vi "Log Level.vi"(8 "error in (no error)":errorcluster, 11 "Configuration.Level":T1) -> (0 "error out":errorcluster)   [LabVIEW 2016, in "Stream Log.lvlib" / "Global Application Log.lvclass"]
doc: "--\nCopyright © 2017 Composed SystemsI All rights reserved.\n\nAuthor: Jon McBee <jon.mcbee@composed.io>\n\nThis library is provided \"AS IS\" ,WITHOUT WARRANTIES OR\nCONDITIONS OF ANY KIND, either express or implied.\n\nComposed Systems -- composed.io\n\nStream 0.0.1.1\nJon McBee - Composed Systems\nCopyright (c) 2017, Composed Systems"
uses:
  <userlib>/Composed Systems/Stream/Log/Global Application Log/Global Application Log.lvclass
  <userlib>/Composed Systems/Stream/Log/Application Log/Log Level.ctl
  <userlib>/Composed Systems/Stream/Log/Global Application Log/Global Application Log.lvclass/Global Application Log.ctl
  <userlib>/Composed Systems/Stream/Log/Application Log/Application Log.lvclass
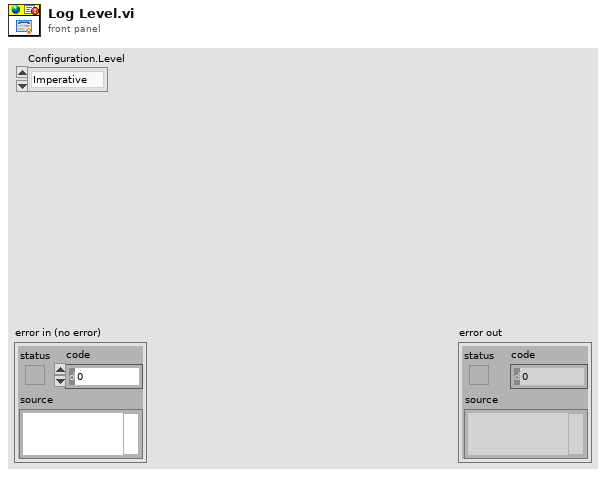
[diagram p1: front panel]
types:
  T1 = typedef "Stream Log.lvlib/Application Log.lvclass/Log Level.ctl" = enum16{"Imperative", "Major", "Minor", "Debug", "Off"}
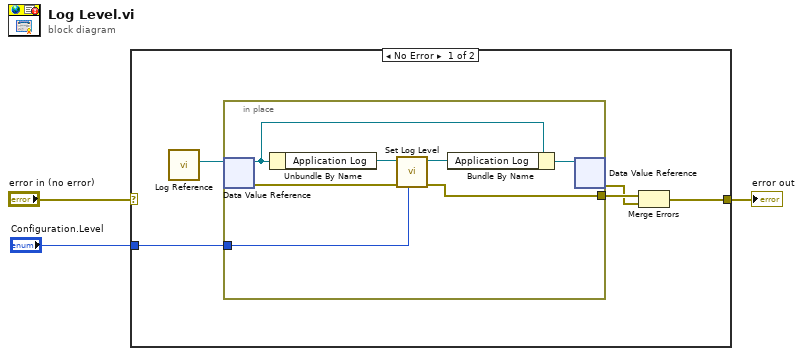
[diagram p0: block diagram]
diagram:
  n1 = case shown="No Error" "error in (no error)" {
    selector: "error in (no error)" -> [_ w16]
    tunnel: [w5 w16] -> w2
    tunnel: "Configuration.Level" -> [w4 _]
    frame No Error {
      n2 = call <userlib>:"Log Reference.vi"() -> ("Global Log Reference out"=w8:refnum<data-value>)  [unwired: 11 in]
      n3 = in-place {
        in-place-border: [w10] -> w7
        in-place-border: w4 -> [w9]
        n4 = in-place-dvr #1(w8) -> (w15:refnum<class "Global Application Log.lvclass">, w11:errorcluster)
        n5 = Unbundle By Name(w15) -> ("Application Log"=w13:refnum<class "Application Log.lvclass">)
        n6 = call <userlib>:"Set Log Level.vi"("Configuration.Level"=w9, "error in (no error)"=w11, "Application Log in"=w13) -> ("error out"=w10:errorcluster, "Application Log out"=w12:refnum<class "Application Log.lvclass">)  [unwired: 7 in]
        n7 = Bundle By Name(cluster=w15, "Application Log"=w12) -> (w14:refnum<class "Global Application Log.lvclass">)
        n8 = in-place-dvr #1(w14) -> (w6:errorcluster)  [unwired: 1 out]
      }
      n9 = Merge Errors(w7, w6) -> (w5:errorcluster)
    }
    frame Error {
    }
  }
  "error out" <- w2
